vi "Inclinometer Output Range.vi"(11 "Data In":T1) -> (3 "Data Out":T1)   [LabVIEW 2018]
doc: "Assert Component\nAssert Name: Inclinometer Output Range\nData Type: Double Float\nDeveloped by Delacor\nEvaluation String: X > 0.500000\nDescription:"
uses:
  Users/Delacor/Documents/LabVIEW Data/Assert API Support/Templates/NC Templates/dbl.ctl
  <vilib>/Assert API/Core/Assert API Components/Failure Actions.ctl
  <vilib>/Assert API/Core/Assert API Components/Assert API Components.lvlib
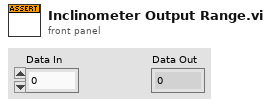
[diagram p1: front panel]
types:
  T1 = typedef "dbl.ctl" = dbl
  T2 = typedef "Assert API Components.lvlib/Failure Actions.ctl" = enum16{"None", "Log To File", "Pause Execution", "Abort Execution"}
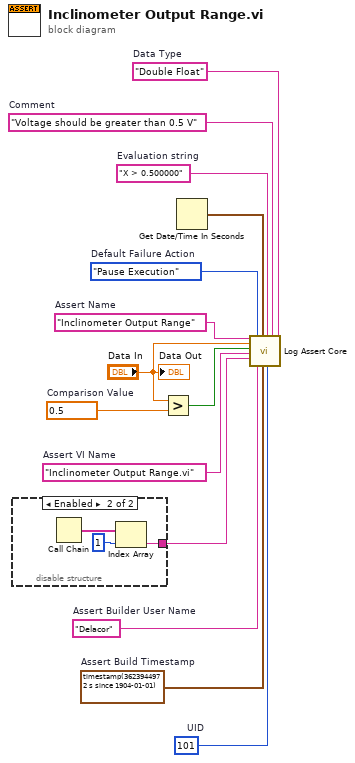
[diagram p0: block diagram]
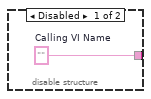
[diagram p2: hidden frame]
diagram:
  w2 = 101  # UID
  w4 = "Inclinometer Output Range.vi"  # Assert VI Name
  w5 = timestamp(3623944972.8137074 s since 1904-01-01)  # Assert Build Timestamp
  w6 = "Delacor"  # Assert Builder User Name
  w7 = "Double Float"  # Data Type
  w11 = "Voltage should be greater than 0.5 V"  # Comment
  w8 = "X > 0.500000"  # Evaluation string
  w13 = Failure_Actions."Pause Execution"  # Default Failure Action
  w14 = "Inclinometer Output Range"  # Assert Name
  w12 = T1 0.5  # Comparison Value
  n1 = disable-structure shown="Enabled" {
    disable-tunnel: [w15 w16] -> w1
    frame Disabled {
      w15 = ""  # Calling VI Name
    }
    frame Enabled {
      n2 = Call Chain() -> (call chain=w17:string[])
      n3 = Index Array(array=w17, index=1) -> (element=w16:string)
    }
  }
  n4 = Greater?(x="Data In", y=w12) -> (0:w9:bool)
  n5 = Get Date/Time In Seconds() -> (seconds since 1Jan1904=w3:timestamp)
  n6 = call <vilib>:"Log Assert Core.vi"("Assert Name"=w14, "Data Value"="Data In", "Status"=w9, "Assert VI Name"=w4, "Calling VI Name"=w1, "Failure Action"=w13, "Assert Builder User Name"=w6, "Last Update"=w3, "Assert Build Timestamp"=w5, "Evaluation String"=w8, "Assert VI UID"=w2, "Comment"=w11, "Data Type"=w7) -> ()  [unwired: 7 in]
  "Data Out" <- "Data In"
